vi "TS DotStar SPI V4.vi"() -> ()   [LabVIEW 2015]
doc: "ADXL362 SPI Accelerometer\n\nThis example shows how to use the Analog Devices ADXL362 Accelerometer sensor connected to SPI.\n\nThis example expects a USB cable connected from your development PC to the Type B USB Jack (next to the power input) on the roboRIO."
uses:
  <vilib>/Rock Robotics/SystemInterfaces/spilib/spi_bus.ctl
  <vilib>/Rock Robotics/WPI/SPI/WPI_SPIMode.ctl
panel:
  out "Aiming 2":bool
  out "Aiming":bool
  out "Intake":bool
  out "Shooter":bool
  in  "Slide":u8(slide) max=31 scale=0.0..31.0
  in  "Numeric 3":u8
  in  "Numeric 2":u8
  in  "Numeric":u8
  in  "Blue":bool
  in  "Red":bool
  in  "Green":bool
  in  "Number of Lights":u8
  in  "Number ON":u8
  in  "Chip Select Active High (F)":bool
  in  "Mode (3)":T1=enum."Mode 3 (Clk Idle High,Sample on Trailing)"
  in  "Clock Rate (Hz)":dbl=500000.0
  in  "error in":errorcluster
  in  "SPI Bus":T2=enum."SPI On-Board, CS1"
  out "error out":errorcluster
  in  "stop":bool
  # "Set these inputs before running."
  # "Number of Lights"
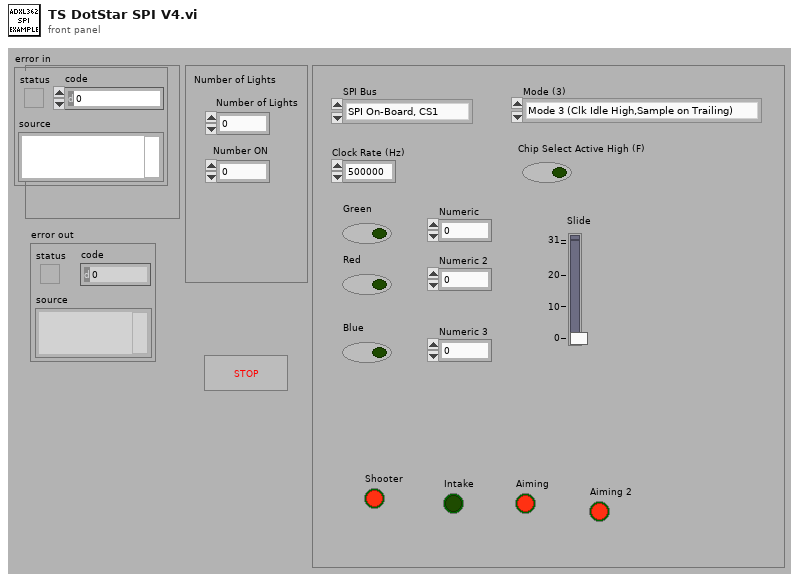
[diagram p1: front panel]
types:
  T1 = typedef "WPI_SPIMode.ctl" = enum16{"Mode 0 (Clk Idle Low,Sample on Leading)", "Mode 1 (Clk Idle Low,Sample on Trailing)", "Mode 2 (Clk Idle High,Sample on Leading)", "Mode 3 (Clk Idle High,Sample on Trailing)"}
  T2 = typedef "spi_bus.ctl" = enum16{"SPI On-Board, CS0", "SPI On-Board, CS1", "SPI On-Board, CS2", "SPI On-Board, CS3", "SPI MXP", "Invalid"}
  T3 = typedef "WPI_SPIDevRef.ctl" = cluster{"DevStatus":errorcluster, "Handle":i32, "SPI Bus":T2}
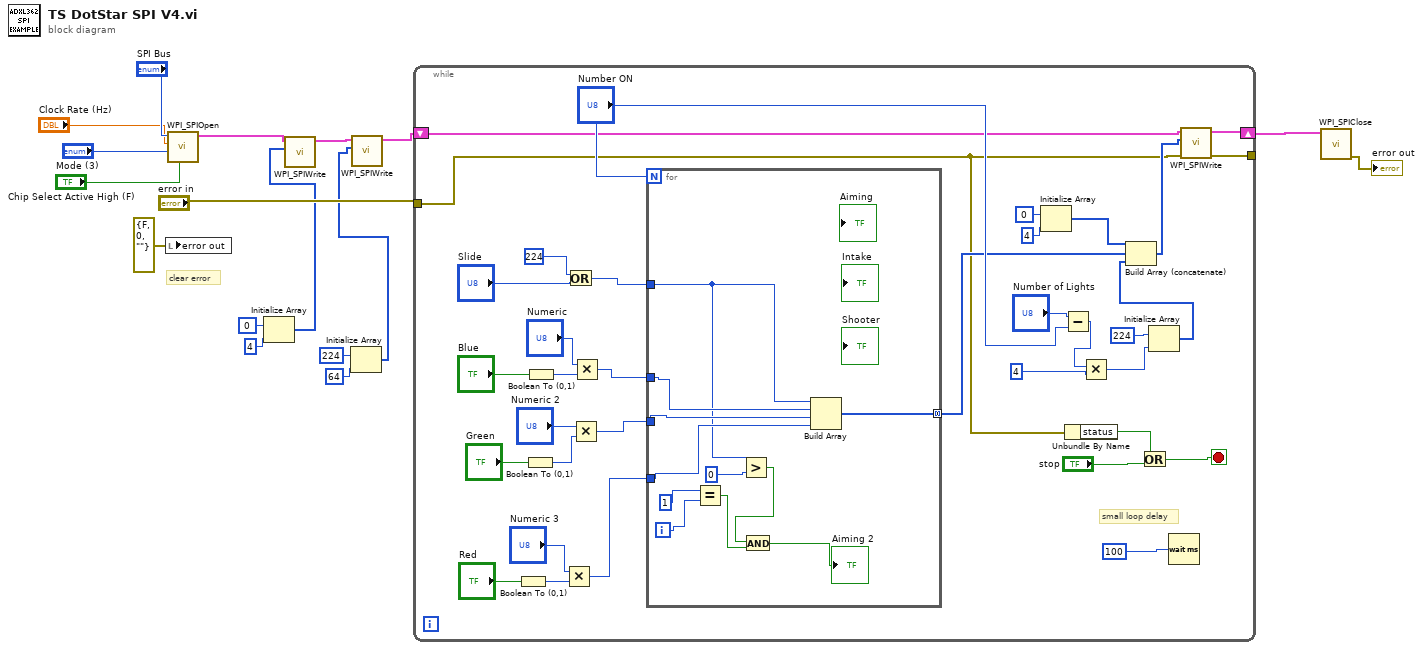
[diagram p0: block diagram]
diagram:
  # "clear error"
  n1 = local write "error out"(errorcluster {"status"=FALSE, "code"=0, "source"=""} ("error out")) -> ()
  n2 = call <vilib>:"WPI_SPIOpen.vi"("Chip Select Active High (F)"="Chip Select Active High (F)", "Mode (3)"="Mode (3)", "Clock Rate (Hz)"="Clock Rate (Hz)", "SPI Bus"="SPI Bus") -> ("SPIDevRef"=w7:T3)  [unwired: 6 in, 1 out]
  n3 = Initialize Array(u8 0 ("Data To Send"), u8 4 ("dimension size")) -> (w6:u8[])
  n4 = call <vilib>:"WPI_SPIWrite.vi"("Data To Send"=w6, "SPIDevRef"=w7) -> ("SPIDevRef"=w5:T3)  [unwired: 7 in, 2 out]
  n5 = Initialize Array(u8 224 ("Data To Send"), u8 64 ("dimension size")) -> (w1:u8[])
  n6 = call <vilib>:"WPI_SPIWrite.vi"("Data To Send"=w1, "SPIDevRef"=w5) -> ("SPIDevRef"=w4:T3)  [unwired: 7 in, 2 out]
  n7 = while {
    shift-right: [w47] -> w14
    shift-left: w4 -> [w25]
    tunnel: "error in" -> [w19]
    tunnel: [w46] -> _
    stop <- w18 stop-if-true
    # "small loop delay"
    n8 = Boolean To (0,1)(Boolean="Red") -> (0, 1=w39:i16)
    n9 = Boolean To (0,1)(Boolean="Green") -> (0, 1=w40:i16)
    n10 = Boolean To (0,1)(Boolean="Blue") -> (0, 1=w41:i16)
    n11 = Multiply(x="Numeric 3", y=w39) -> (x*y=w33:i16)
    n12 = Or(x=u8 224, y="Slide") -> (x .or. y?=w30:u8)
    n13 = Multiply(x="Numeric 2", y=w40) -> (x*y=w34:i16)
    n14 = Multiply(x="Numeric", y=w41) -> (x*y=w35:i16)
    n15 = for {
      N: "Number ON" -> [_]
      tunnel: w35 -> [w63]
      tunnel: w34 -> [w62]
      tunnel: w33 -> [w61]
      tunnel: w30 -> [w56]
      tunnel: [w60] -> w23 mode=concatenating
      i -> [w59]
      n16 = Equal?(x=u8 1 ("dimension size"), y=w59) -> (x = y?=w57:bool)
      n17 = Greater?(x=w56, y=u8 0 ("dimension size")) -> (0:w54:bool)
      n18 = And(x=w54, y=w57) -> (x .and. y?=→"Aiming 2":bool)
      n19 = Build Array(w56, w63, w62, w61) -> (w60:i16[])
    }
    n20 = Initialize Array(u8 0 ("Data To Send"), u8 4 ("dimension size")) -> (w24:u8[])
    n21 = Subtract(x="Number of Lights", y="Number ON") -> (x-y=w26:u8)
    n22 = Unbundle By Name(w19) -> ("status"=w20:bool)
    n23 = Multiply(x=w26, y=u8 4 ("dimension size")) -> (x*y=w29:u8)
    n24 = Or(x=w20, y="stop") -> (x .or. y?=w18:bool)
    n25 = Initialize Array(u8 224 ("Data To Send"), w29) -> (w22:u8[])
    n26 = Build Array (concatenate)(w24, w23, w22) -> (w21:i16[])
    n27 = Wait (ms)(milliseconds to wait=u32 100) -> ()  [unwired: 1 out]
    n28 = call <vilib>:"WPI_SPIWrite.vi"("error in (no error)"=w19, "Data To Send"=w21, "SPIDevRef"=w25) -> ("error out"=w46:errorcluster, "SPIDevRef"=w47:T3)  [unwired: 6 in, 1 out]
  }
  n29 = call <vilib>:"WPI_SPIClose.vi"("SPIDevRef"=w14) -> ("error out"=→"error out":errorcluster)  [unwired: 10 in]
